vi "3.3 Building Virtual Instruments-Lab1(Prob2).vi"() -> ()   [LabVIEW 2025]
panel:
  in  "stop":bool
  out "Degree in Fahrenheit":dbl
  in  "Degrees in Celsius":dbl
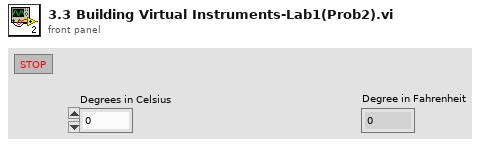
[diagram p1: front panel]
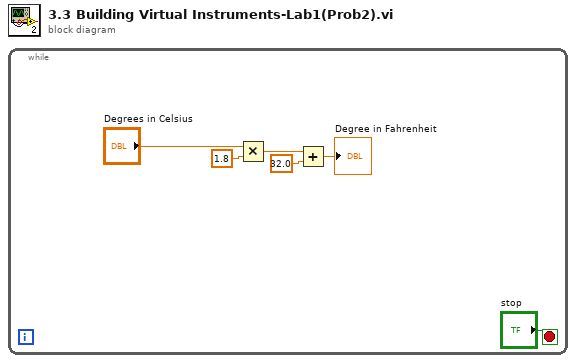
[diagram p0: block diagram]
diagram:
  n1 = while {
    stop <- "stop" stop-if-true
    n2 = Multiply(x="Degrees in Celsius", y=1.8) -> (x*y=w4:dbl)
    n3 = Add(x=w4, y=32.0) -> (x+y=→"Degree in Fahrenheit":dbl)
  }
